vi "Transfer ID to Tree Items.vi"(8 "error in (no error)":errorcluster, 9 "Transfer ID":string, 11 "Application Data in":T2) -> (0 "error out":errorcluster, 1 "Settings":T1, 2 "Item":T1, 3 "Application Data out":T2)   [LabVIEW 2017, in "DSF Data Viewer.lvlib"]
uses:
  DSF Data Viewer.lvlib
  Main VI/Application Data.ctl
  Builds/Data Sharing Framework/Current/Core/DSF Core.lvlibp/Engine/Classes/Framework/Framework.lvclass
  <vilib>/NI/Memory Manager/Classes/Pointer/Pointer.lvclass
  Buffer Reader/Buffer Data.ctl
  Builds/Data Sharing Framework/Current/Core/DSF Core.lvlibp/Engine/Classes/Buffer/Buffer.lvclass
  Tree Item.ctl
  Tree Item Type.ctl
  Builds/Data Sharing Framework/Current/Core/DSF Core.lvlibp/DSF Configuration API/Configuration Session.lvclass
  Builds/Data Sharing Framework/Current/Core/DSF Core.lvlibp/DSF Configuration API/Public/Read Item/Read Settings.vi
  Builds/Data Sharing Framework/Current/Core/DSF Core.lvlibp/DSF Configuration API/Public/Read Item/Read Transfer.vi
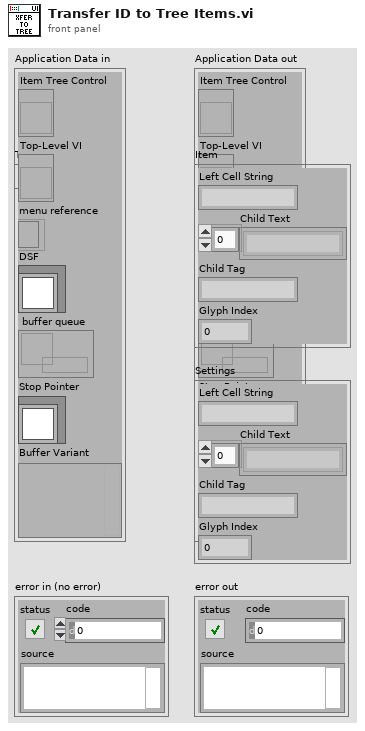
[diagram p1: front panel]
types:
  T1 = typedef "DSF Data Viewer.lvlib/Tree Item.ctl" = cluster{"Left Cell String":string, "Child Text":string[], "Child Tag":string, "Glyph Index":i32}
  T2 = typedef "DSF Data Viewer.lvlib/Application Data.ctl" = cluster{"Item Tree Control":refnum<vi>, "Top-Level VI":refnum<vi>, "menu reference":refnum<k9>, "DSF":refnum<class "Framework.lvclass">, "buffer queue":refnum<queue>, "Stop Pointer":refnum<class "Pointer.lvclass">, "Buffer Variant":variant}
  T3 = typedef "DSF Data Viewer.lvlib/Tree Item Type.ctl" = enum16{"Framework", "Plugin Group", "Plugin", "Group", "Transfer", "Buffer", "Channel"}
  T4 = typedef "DSF Core.lvlibp/DSF Transfer Info.ctl" = cluster{"byte order":T5, "channel ids":string[], "settings id":string}
  T5 = typedef "DSF Core.lvlibp/DSF Byte Order.ctl" = enum8{"big-endian", "little-endian"}
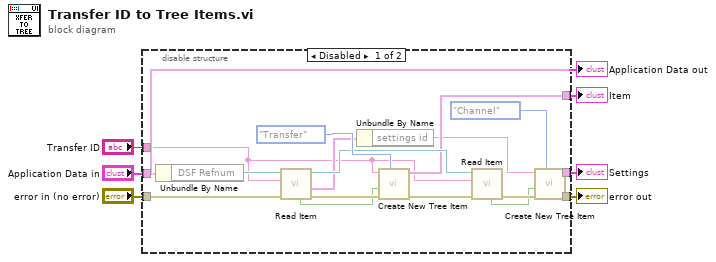
[diagram p0: block diagram]
diagram:
  n1 = disable-structure shown="Disabled" {
    disable-tunnel: "error in (no error)" -> [w18 _]
    disable-tunnel: [w15 _] -> w5
    disable-tunnel: "Application Data in" -> [w13 _]
    disable-tunnel: [w12 _] -> w3
    disable-tunnel: [w11 _] -> w2
    disable-tunnel: "Transfer ID" -> [w7 _]
    frame Disabled {
      n2 = Unbundle By Name(w13) -> ("DSF Refnum"=w14:refnum<class "Configuration Session.lvclass">)
      n3 = call-poly "Read Item.vi"("error in (no error)"=w18, "Transfer ID"=w7, "Configuration Session in"=w14) -> ("error out"=w19:errorcluster, "value"=w16:T4, "Configuration Session out"=w17:refnum<class "Configuration Session.lvclass">, "found?"=w8:bool)  [unwired: 5 in]
      n4 = Unbundle By Name(w16) -> ("settings id"=w10:string)
      n5 = call "Create New Tree Item.vi"("Item Type"=Tree_Item_Type."Transfer", "error in"=w19, "found?"=w8, "Left Cell String"=w7) -> ("error out"=w20:errorcluster, "Item"=w12:T1)  [unwired: 6 in]
      n6 = call-poly "Read Item.vi"("error in (no error)"=w20, "Settings ID"=w7, "Configuration Session in"=w17) -> ("error out"=w21:errorcluster, "found?"=w9:bool)  [unwired: 5 in, 2 out]
      n7 = call "Create New Tree Item.vi"("Item Type"=Tree_Item_Type."Channel", "error in"=w21, "found?"=w9, "Left Cell String"=w10) -> ("error out"=w15:errorcluster, "Item"=w11:T1)  [unwired: 6 in]
    }
    frame Enabled {
    }
  }
  "error out" <- w5
  "Item" <- w3
  "Settings" <- w2
  "Application Data out" <- "Application Data in"
